vi "Servo main.vi"(8 "Queue to UI":T1, 11 "Module queue servo":T1) -> ()   [LabVIEW 2024, in "Servo drive module.lvlib"]
doc: "This is TOP VI for Servo control.\n\nCommands:\nInitialize ( ) - Open connections to drivers by ethernet, and gets \nUpdate( ) - Get actual position and makes calculations if something changed\nMove(relative position, axis) - moves by defined step\nEnd( )\n\nResponses: \nStatus changed (quick status[IP addr, Connection, connected, Name, powered, act pos., desir. pos.])\nInitialized (status[connected, powered, act pos., desir. pos.])\nError ... (error cluster) - adds \"error\" before casual response"
uses:
  Servo drive module.lvlib
  Messenger service/Data types/Mailbox address.ctl
  ctl/Servo state.ctl
  ctl/Servo variables.ctl
  ctl/Servo constants.ctl
  ctl/Axis names.ctl
  ctl/Servo MSG.ctl
  ctl/Servo commands.ctl
  Messenger service/Data types/Module name.ctl
  <vilib>/addons/eal4LabVIEW/eal4LabVIEW.lvlib
  Messenger service/MessengerLib.lvlib
panel:
  out "Error out":errorcluster
  out "Ended":bool
  out "Connected":bool
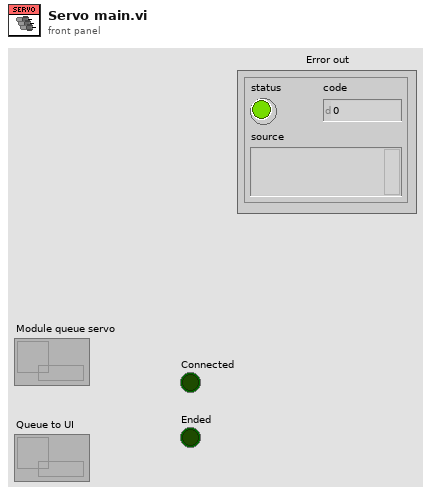
[diagram p1: front panel]
types:
  T1 = typedef "MessengerLib.lvlib/Mailbox address.ctl" = refnum<queue>
  T2 = typedef "Servo drive module.lvlib/Servo state.ctl" = cluster{"Servo variables":T3, "Servo constants":T4, "Connection":variant}
  T3 = typedef "Servo drive module.lvlib/Servo variables.ctl" = cluster{"Terget reached":bool, "Connected":bool, "Power ON":bool, "Operation mode":bool, "Actual position":dbl, "Target position":dbl}
  T4 = typedef "Servo drive module.lvlib/Servo constants.ctl" = cluster{"Name":T5, "Pos position limit [mm]":dbl, "Neg position limit [mm]":dbl, "Pos velocity limit":dbl, "Neg velocity limit":dbl, "Acceleration limit":dbl}
  T5 = typedef "Servo drive module.lvlib/Axis names.ctl" = enum16{"Unknown", "AxisX", "AxisY", "AxisZ_left", "AxisZ_middle", "AxisZ_right"}
  T6 = typedef "Module name.ctl" = enum16{"Emty", "Magnet", "VTI", "Excitation", "Servo", "Acquisition", "Rotator", "Digitizer", "SMU2450", "Carousel", "Multimeter", "Tmp monitor", "Power monitor"}
  T7 = typedef "Servo drive module.lvlib/Servo MSG.ctl" = cluster{"Command":T8, "Data":variant}
  T8 = typedef "Servo drive module.lvlib/Servo commands.ctl" = enum16{"Initialize", "Update", "Move by", "Move to", "Stop", "Ignore", "Disconnect", "End"}
  T9 = typedef "Servo drive module.lvlib/Status variable change.ctl" = cluster{"Property":string, "Value":variant, "Name":T5}
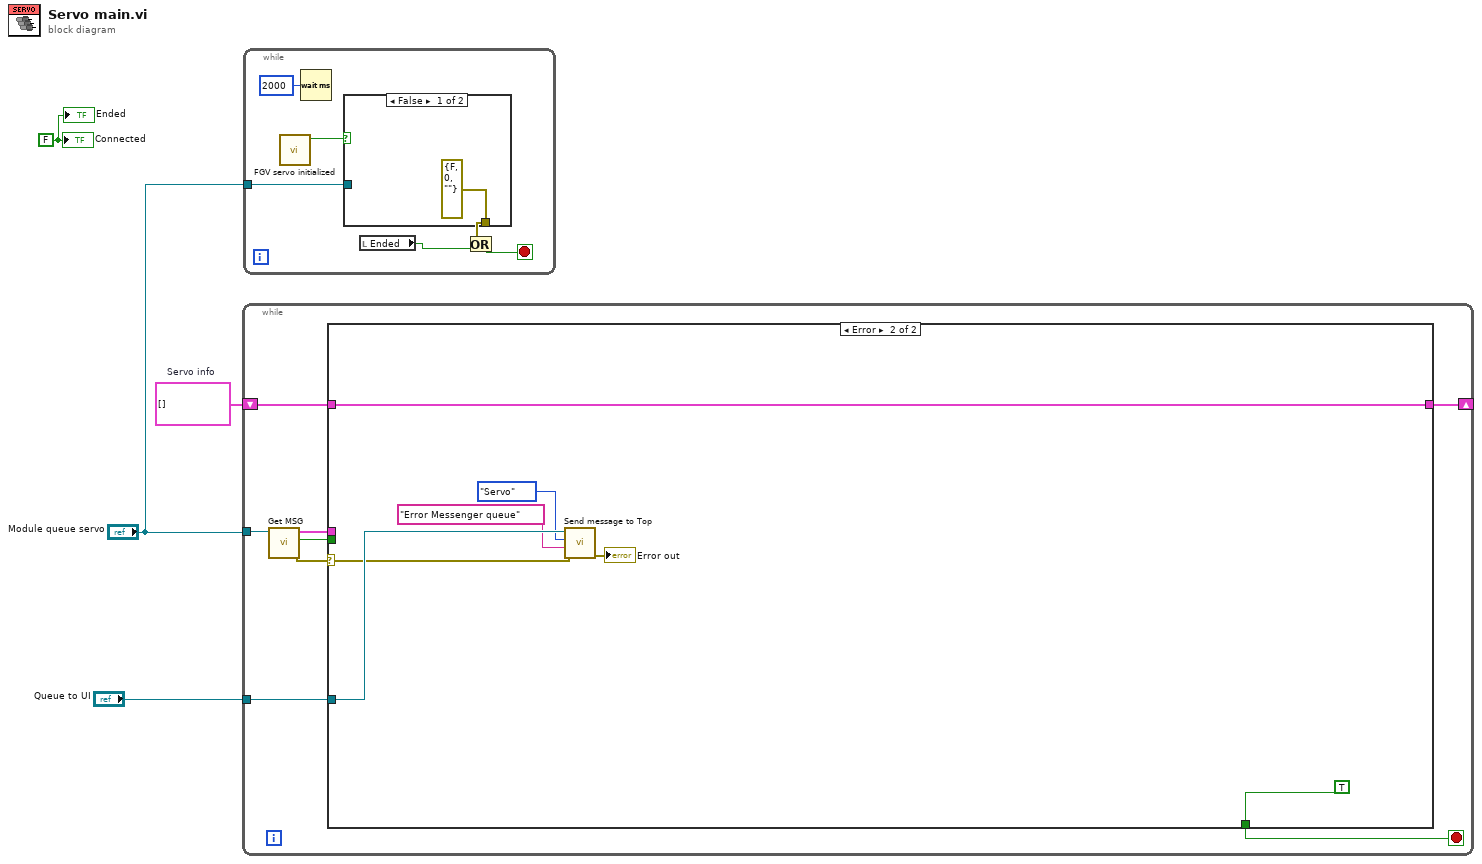
[diagram p0: block diagram]
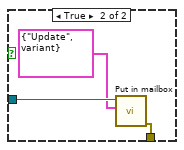
[diagram p2: hidden frame]
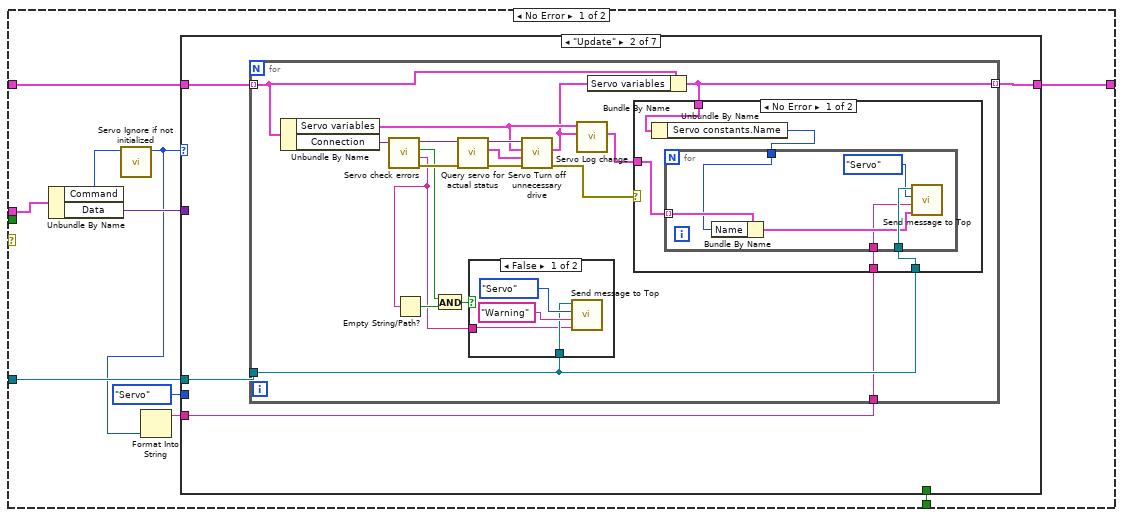
[diagram p3: hidden frame]
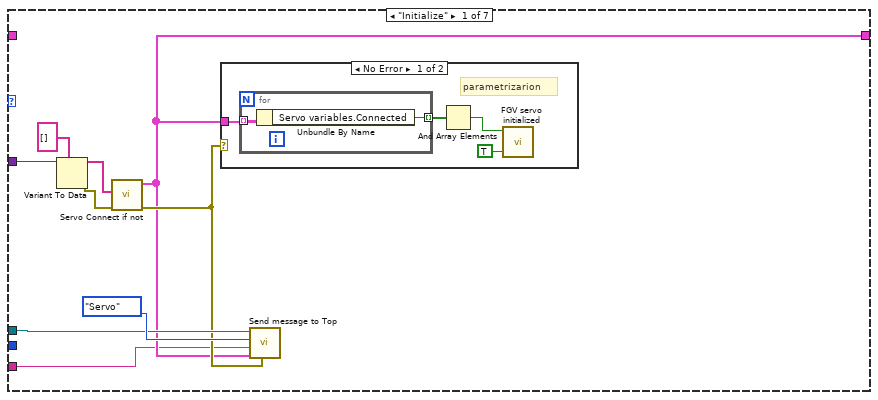
[diagram p4: hidden frame]
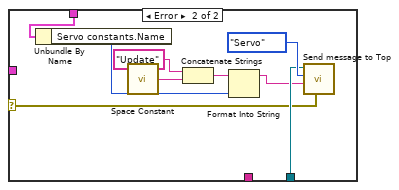
[diagram p7: hidden frame]
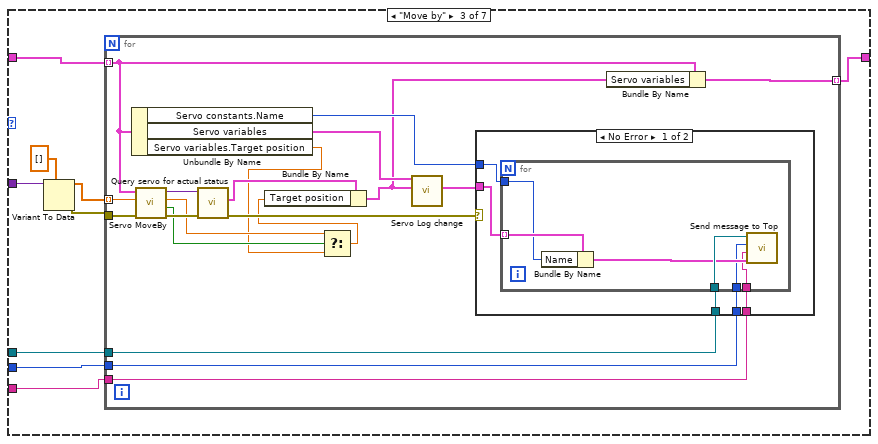
[diagram p8: hidden frame]
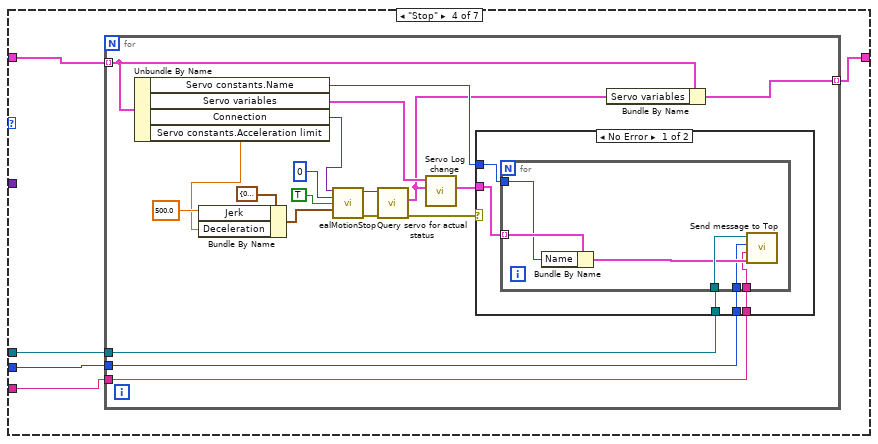
[diagram p10: hidden frame]
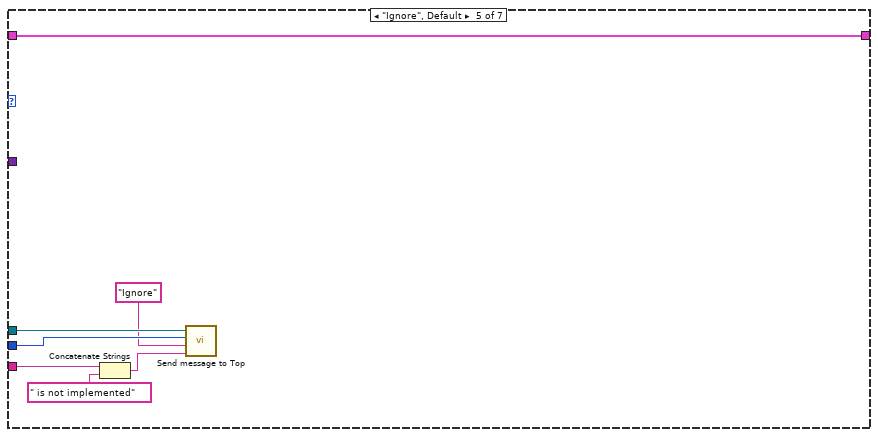
[diagram p12: hidden frame]
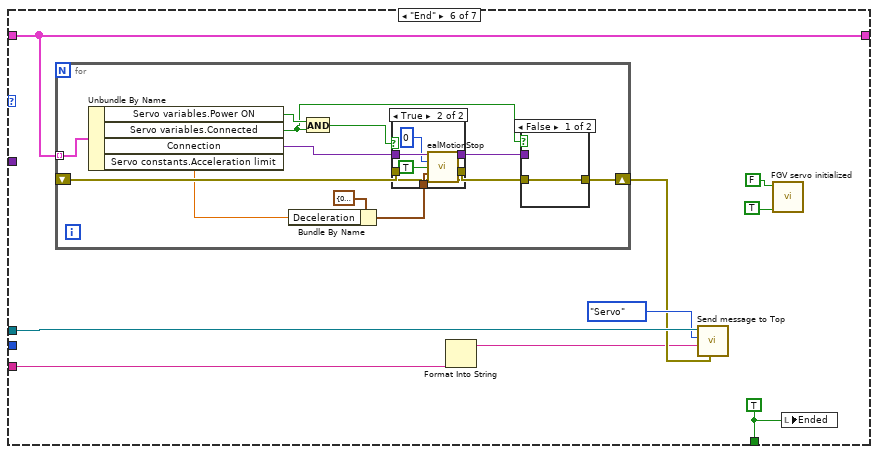
[diagram p13: hidden frame]
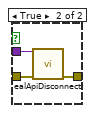
[diagram p14: hidden frame]
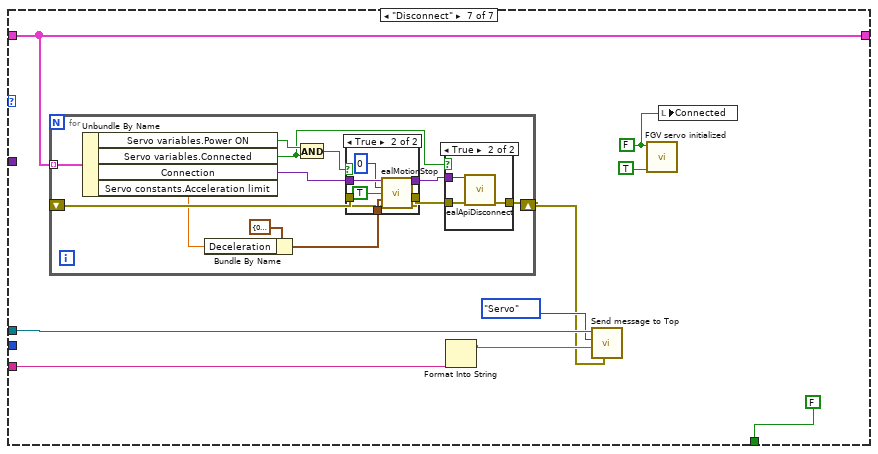
[diagram p16: hidden frame]
diagram:
  w1 = FALSE ("Initialized in")
  w3 = T2[] []  # Servo info
  n1 = while {
    tunnel: "Queue to UI" -> [w12]
    tunnel: "Module queue servo" -> [w11]
    shift-right: [w9] -> _
    shift-left: w3 -> [w10]
    stop <- w6 stop-if-true
    n2 = call "Get MSG.vi"("Queue in"=w11) -> ("error out"=w5:errorcluster, "more than five"=w8:bool, "MSG for servo"=w7:T7)  [unwired: 8 in]
    n3 = case shown="Error" w5 {
      selector: w5 -> [_ w234]
      tunnel: w8 -> [_ _]
      tunnel: w7 -> [w22 _]
      tunnel: w10 -> [w20 w236]
      tunnel: [w19 w236] -> w9
      tunnel: w12 -> [w18 w239]
      tunnel: [w16 TRUE] -> w6
      frame No Error {
        n4 = Unbundle By Name(w22) -> ("Command"=w17:T8, "Data"=w21:variant)
        n5 = call "Servo Ignore if not initialized.vi"("Command in"=w17) -> ("command out"=w13:T8)  [unwired: 10 in]
        n6 = Format Into String(w13) -> (resulting string=w14:string)  [unwired: 3 in, 1 out]
        n7 = case shown="\"Update\"" w13 {
          tunnel: w21 -> [w27 _ w89 _ _ _ _]
          tunnel: w20 -> [_ w41 w91 w126 w164 w171 w200]
          tunnel: [w28 w40 w90 w125 w164 w171 w200] -> w19
          tunnel: w18 -> [w30 w39 w92 w127 w163 w170 w205]
          tunnel: [_ _ _ _ _ w165 FALSE] -> w16
          tunnel: Module_name."Servo" ("Module") -> [_ _ w85 w124 w162 _ _]
          tunnel: w14 -> [w23 w38 w84 w123 w159 w166 w202]
          frame "Initialize" {
            n8 = Variant To Data(type=string[] [], Variant=w27) -> (data=w25:string[], error out=w24:errorcluster)  [unwired: 1 in]
            n9 = call "Servo Connect if not.vi"("error in"=w24, "IP addresses"=w25) -> ("error out"=w29:errorcluster, "Servo statuses"=w28:T2[])  [unwired: 8 in]
            n10 = case shown="No Error" w29 {
              tunnel: w28 -> [w33 _]
              frame No Error {
                # "parametrizarion"
                n11 = for {
                  tunnel: w33 -> [w37] mode=indexing
                  tunnel: [w36] -> w32 mode=indexing
                  n12 = Unbundle By Name(w37) -> ("Servo variables.Connected"=w36:bool)
                }
                n13 = And Array Elements(Boolean array=w32) -> (logical AND=w34:bool)
                n14 = call "FGV servo initialized.vi"("Write?(F)"=TRUE, "Initialized in"=w34) -> ()  [unwired: 9 in, 1 out]
              }
              frame Error {
              }
            }
            n15 = call "Send message to Top.vi"("Error in (no error)"=w29, "Data"=w28, "Response"=w23, "Module"=Module_name."Servo", "Mailbox address in"=w30) -> ()  [unwired: 5 in, 2 out]
          }
          frame "Update" {
            n16 = for {
              tunnel: w39 -> [w52]
              tunnel: w41 -> [w49] mode=indexing
              tunnel: [w47] -> w40 mode=indexing
              tunnel: w38 -> [w42]
              n17 = Unbundle By Name(w49) -> ("Servo variables"=w46:T3, "Connection"=w56:variant)
              n18 = call "Servo check errors.vi"("connection in"=w56) -> ("error out"=w58:errorcluster, "diagnosis text"=w53:string, "OK"=w57:bool, "connection out"=w51:variant)  [unwired: 7 in]
              n19 = Empty String/Path?(string/path=w53) -> (empty?=w54:bool)
              n20 = And(x=w57, y=w54) -> (x .and. y?=w55:bool)
              n21 = call "Query servo for actual status.vi"("error in (no error)"=w58, "connection in"=w51) -> ("error out"=w59:errorcluster, "Servo variables"=w48:T3, "connection out"=w50:variant)  [unwired: 7 in]
              n22 = case shown="False" w55 {
                tunnel: w52 -> [w61 _]
                tunnel: w53 -> [w60 _]
                frame False {
                  n23 = call "Send message to Top.vi"("Data"=w60, "Response"="Warning", "Module"=Module_name."Servo", "Mailbox address in"=w61) -> ()  [unwired: 6 in, 2 out]
                }
                frame True {
                }
              }
              n24 = call "Servo Turn off unnecessary drive.vi"("error in (no error)"=w59, "Status now"=w48, "Status before"=w46, "Connection"=w50) -> ("error out"=w45:errorcluster, "Status out"=w43:T3)  [unwired: 6 in]
              n25 = call "Servo Log change.vi"("Servo variables Now"=w43, "Servo variables Before"=w46) -> ("Changes"=w44:T9[])  [unwired: 8 in, 1 out]
              n26 = Bundle By Name(cluster=w49, "Servo variables"=w43) -> (w47:T2)
              n27 = case shown="No Error" w45 {
                selector: w45 -> [_ w80]
                tunnel: w52 -> [w67 w81]
                tunnel: w47 -> [w66 w79]
                tunnel: w44 -> [w68 _]
                tunnel: w42 -> [w64 _]
                frame No Error {
                  n28 = Unbundle By Name(w66) -> ("Servo constants.Name"=w65:T5)
                  n29 = for {
                    tunnel: w68 -> [w72] mode=indexing
                    tunnel: w67 -> [w74]
                    tunnel: w65 -> [w70]
                    tunnel: w64 -> [w69]
                    n30 = Bundle By Name(cluster=w72, "Name"=w70) -> (w71:T9)
                    n31 = call "Send message to Top.vi"("Data"=w71, "Response"=w69, "Module"=Module_name."Servo", "Mailbox address in"=w74) -> ()  [unwired: 6 in, 2 out]
                  }
                }
                frame Error {
                  n32 = Unbundle By Name(w79) -> ("Servo constants.Name"=w77:T5)
                  n33 = call <vilib>:"Space Constant.vi"() -> ("String"=w83:string)
                  n34 = Concatenate Strings("Update" ("Response"), w83) -> (w76:string)
                  n35 = Format Into String(initial string=w76, w77) -> (resulting string=w75:string)  [unwired: 2 in, 1 out]
                  n36 = call "Send message to Top.vi"("Error in (no error)"=w80, "Response"=w75, "Module"=Module_name."Servo", "Mailbox address in"=w81) -> ()  [unwired: 6 in, 2 out]
                }
              }
            }
          }
          frame "Move by" {
            n37 = Variant To Data(type=dbl[] [], Variant=w89) -> (data=w88:dbl[], error out=w86:errorcluster)  [unwired: 1 in]
            n38 = for {
              tunnel: w92 -> [w111]
              tunnel: w88 -> [w110] mode=indexing
              tunnel: w91 -> [w109] mode=indexing
              tunnel: [w108] -> w90 mode=indexing
              tunnel: w86 -> [w96]
              tunnel: w85 -> [w95]
              tunnel: w84 -> [w94]
              n39 = Unbundle By Name(w109) -> ("Servo constants.Name"=w105:T5, "Servo variables"=w107:T3, "Servo variables.Target position"=w97:dbl)
              n40 = call "Servo MoveBy.vi"("error in"=w96, "Move by"=w110, "Status in"=w109) -> ("error out"=w104:errorcluster, "executed"=w100:bool, "Target position"=w99:dbl, "connection out"=w101:variant)  [unwired: 5 in]
              n41 = call "Query servo for actual status.vi"("error in (no error)"=w104, "connection in"=w101) -> ("error out"=w103:errorcluster, "Servo variables"=w102:T3)  [unwired: 7 in, 1 out]
              n42 = Select(t=w99, s=w100, f=w97) -> (s? t:f=w98:dbl)
              n43 = Bundle By Name(cluster=w102, "Target position"=w98) -> (w93:T3)
              n44 = call "Servo Log change.vi"("Servo variables Now"=w93, "Servo variables Before"=w107) -> ("Changes"=w106:T9[])  [unwired: 8 in, 1 out]
              n45 = case shown="No Error" w103 {
                tunnel: w111 -> [w116 _]
                tunnel: w106 -> [w115 _]
                tunnel: w105 -> [w114 _]
                tunnel: w95 -> [w113 _]
                tunnel: w94 -> [w112 _]
                frame No Error {
                  n46 = for {
                    tunnel: w116 -> [w122]
                    tunnel: w115 -> [w121] mode=indexing
                    tunnel: w114 -> [w119]
                    tunnel: w113 -> [w118]
                    tunnel: w112 -> [w117]
                    n47 = Bundle By Name(cluster=w121, "Name"=w119) -> (w120:T9)
                    n48 = call "Send message to Top.vi"("Data"=w120, "Response"=w117, "Module"=w118, "Mailbox address in"=w122) -> ()  [unwired: 6 in, 2 out]
                  }
                }
                frame Error {
                }
              }
              n49 = Bundle By Name(cluster=w109, "Servo variables"=w93) -> (w108:T2)
            }
          }
          frame "Stop" {
            n50 = for {
              tunnel: w127 -> [w146]
              tunnel: w126 -> [w132] mode=indexing
              tunnel: [w145] -> w125 mode=indexing
              tunnel: w124 -> [w140]
              tunnel: w123 -> [w139]
              n51 = Unbundle By Name(w132) -> ("Servo constants.Name"=w142:T5, "Servo variables"=w144:T3, "Connection"=w129:variant, "Servo constants.Acceleration limit"=w128:dbl)
              n52 = Bundle By Name(cluster=cluster{"Deceleration":dbl, "Jerk":dbl} {"Deceleration"=0.0, "Jerk"=0.0} ("parameters set"), "Jerk"=500.0, "Deceleration"=w128) -> (w136:cluster{"Deceleration":dbl, "Jerk":dbl})
              n53 = call <vilib>:"ealMotionStop.vi"("connection in"=w129, "slave index"=0, "stop"=TRUE, "parameters set"=w136) -> ("connection out"=w135:variant, "error out"=w138:errorcluster)  [unwired: 10 in]
              n54 = call "Query servo for actual status.vi"("error in (no error)"=w138, "connection in"=w135) -> ("error out"=w141:errorcluster, "Servo variables"=w133:T3)  [unwired: 7 in, 1 out]
              n55 = call "Servo Log change.vi"("Servo variables Now"=w133, "Servo variables Before"=w144) -> ("Changes"=w143:T9[])  [unwired: 8 in, 1 out]
              n56 = case shown="No Error" w141 {
                tunnel: w146 -> [w151 _]
                tunnel: w143 -> [w150 _]
                tunnel: w142 -> [w149 _]
                tunnel: w140 -> [w148 _]
                tunnel: w139 -> [w147 _]
                frame No Error {
                  n57 = for {
                    tunnel: w151 -> [w157]
                    tunnel: w150 -> [w156] mode=indexing
                    tunnel: w149 -> [w154]
                    tunnel: w148 -> [w153]
                    tunnel: w147 -> [w152]
                    n58 = Bundle By Name(cluster=w156, "Name"=w154) -> (w155:T9)
                    n59 = call "Send message to Top.vi"("Data"=w155, "Response"=w152, "Module"=w153, "Mailbox address in"=w157) -> ()  [unwired: 6 in, 2 out]
                  }
                }
                frame Error {
                }
              }
              n60 = Bundle By Name(cluster=w132, "Servo variables"=w133) -> (w145:T2)
            }
          }
          frame "Ignore", Default {
            n61 = Concatenate Strings(w159, " is not implemented") -> (w160:string)
            n62 = call "Send message to Top.vi"("Data"=w160, "Response"="Ignore", "Module"=w162, "Mailbox address in"=w163) -> ()  [unwired: 6 in, 2 out]
          }
          frame "End" {
            w165 = TRUE
            n63 = for {
              tunnel: w171 -> [w185] mode=indexing
              shift-right: [w184] -> w168
              shift-left: _ -> [w178]
              n64 = Unbundle By Name(w185) -> ("Servo variables.Power ON"=w176:bool, "Servo variables.Connected"=w174:bool, "Connection"=w183:variant, "Servo constants.Acceleration limit"=w177:dbl)
              n65 = Bundle By Name(cluster=cluster{"Deceleration":dbl, "Jerk":dbl} {"Deceleration"=0.0, "Jerk"=0.0} ("parameters set"), "Deceleration"=w177) -> (w179:cluster{"Deceleration":dbl, "Jerk":dbl})
              n66 = And(x=w176, y=w174) -> (x .and. y?=w175:bool)
              n67 = case shown="True" w175 {
                tunnel: w183 -> [w191 w198]
                tunnel: [w191 w197] -> w182
                tunnel: [w190 w194] -> w181
                tunnel: w179 -> [_ w193]
                tunnel: w178 -> [w190 w192]
                frame False {
                }
                frame True {
                  n68 = call <vilib>:"ealMotionStop.vi"("connection in"=w198, "slave index"=0, "stop"=TRUE, "parameters set"=w193, "error in (no error)"=w192) -> ("connection out"=w197:variant, "error out"=w194:errorcluster)  [unwired: 9 in]
                }
              }
              n69 = case shown="False" w174 {
                tunnel: [w186 w189] -> w184
                tunnel: w182 -> [_ w188]
                tunnel: w181 -> [w186 w187]
                frame False {
                }
                frame True {
                  n70 = call <vilib>:"ealApiDisconnect.vi"("connection in"=w188, "error in (no error)"=w187) -> ("error out"=w189:errorcluster)  [unwired: 13 in]
                }
              }
            }
            n71 = Format Into String(w166) -> (resulting string=w167:string)  [unwired: 3 in, 1 out]
            n72 = call "Send message to Top.vi"("Error in (no error)"=w168, "Response"=w167, "Module"=Module_name."Servo", "Mailbox address in"=w170) -> ()  [unwired: 6 in, 2 out]
            n73 = call "FGV servo initialized.vi"("Write?(F)"=TRUE ("Initialized in"), "Initialized in"=FALSE) -> ()  [unwired: 9 in, 1 out]
            n74 = local write "Ended"(w165) -> ()
          }
          frame "Disconnect" {
            w201 = FALSE ("Initialized in")
            n75 = for {
              tunnel: w200 -> [w219] mode=indexing
              shift-right: [w218] -> w199
              shift-left: _ -> [w212]
              n76 = Unbundle By Name(w219) -> ("Servo variables.Power ON"=w210:bool, "Servo variables.Connected"=w208:bool, "Connection"=w217:variant, "Servo constants.Acceleration limit"=w211:dbl)
              n77 = Bundle By Name(cluster=cluster{"Deceleration":dbl, "Jerk":dbl} {"Deceleration"=0.0, "Jerk"=0.0} ("parameters set"), "Deceleration"=w211) -> (w213:cluster{"Deceleration":dbl, "Jerk":dbl})
              n78 = And(x=w210, y=w208) -> (x .and. y?=w209:bool)
              n79 = case shown="True" w209 {
                tunnel: w217 -> [w225 w232]
                tunnel: [w225 w231] -> w216
                tunnel: [w224 w228] -> w215
                tunnel: w213 -> [_ w227]
                tunnel: w212 -> [w224 w226]
                frame False {
                }
                frame True {
                  n80 = call <vilib>:"ealMotionStop.vi"("connection in"=w232, "slave index"=0, "stop"=TRUE, "parameters set"=w227, "error in (no error)"=w226) -> ("connection out"=w231:variant, "error out"=w228:errorcluster)  [unwired: 9 in]
                }
              }
              n81 = case shown="True" w208 {
                tunnel: [w220 w223] -> w218
                tunnel: w216 -> [_ w222]
                tunnel: w215 -> [w220 w221]
                frame False {
                }
                frame True {
                  n82 = call <vilib>:"ealApiDisconnect.vi"("connection in"=w222, "error in (no error)"=w221) -> ("error out"=w223:errorcluster)  [unwired: 13 in]
                }
              }
            }
            n83 = Format Into String(w202) -> (resulting string=w203:string)  [unwired: 3 in, 1 out]
            n84 = call "Send message to Top.vi"("Error in (no error)"=w199, "Response"=w203, "Module"=Module_name."Servo", "Mailbox address in"=w205) -> ()  [unwired: 6 in, 2 out]
            n85 = call "FGV servo initialized.vi"("Write?(F)"=TRUE ("Initialized in"), "Initialized in"=w201) -> ()  [unwired: 9 in, 1 out]
            n86 = local write "Connected"(w201) -> ()
          }
        }
      }
      frame Error {
        n87 = call "Send message to Top.vi"("Data"=w234, "Response"="Error Messenger queue", "Module"=Module_name."Servo", "Mailbox address in"=w239) -> ("Error out"=→"Error out":errorcluster)  [unwired: 6 in, 1 out]
      }
    }
  }
  n88 = while {
    tunnel: "Module queue servo" -> [w243]
    stop <- w241 stop-if-true
    n89 = call "FGV servo initialized.vi"() -> ("Initialized out"=w244:bool)  [unwired: 11 in]
    n90 = Wait (ms)(milliseconds to wait=u32 2000) -> ()  [unwired: 1 out]
    n91 = case shown="False" w244 {
      tunnel: w243 -> [_ w249]
      tunnel: [errorcluster {"status"=FALSE, "code"=0, "source"=""} ("error out") w248] -> w242
      frame False {
      }
      frame True {
        n92 = call "Put in mailbox.vi"("Message"=T7 {"Command"=enum."Update", "Data"=variant(dbl[] [])} ("MSG to Servo"), "Queue in"=w249) -> ("error out"=w248:errorcluster)  [unwired: 7 in, 2 out]
      }
    }
    n93 = local read "Ended"() -> (w240:bool)
    n94 = Or(x=w242, y=w240) -> (x .or. y?=w241:bool)
  }
  "Connected" <- w1
  "Ended" <- w1
